vi "Retrieve.vi"(8 "error in (no error)":errorcluster, 11 "Error Code":i32) -> (0 "error out":errorcluster, 3 "Filter?":bool)   [LabVIEW 2026, in "TALOS.lvlib" / "Classes.lvlib" / "Error Filter.lvclass"]
doc: "Use this VI to add an error to be skipped in the future. If repetitions and time are both left to zero, the error will be permanently skipped: otherwise the error will be skipped until at least one of the two conditions will be met."
uses:
  Error Filter.lvclass
  Ancestor/Ancestor/Ancestor.lvclass/Ancestor.ctl
  Support VIs/Generate Error.vi
  FGV/Error Memory/Get Error Description.vi
  Support VIs/Get PC name.vi
  Ancestor/Ancestor/Read ID.vi
  Support VIs/Get Class Name.vi
  <vilib>/Utility/error.llb/Clear Errors.vi
  FGV/Error Memory/Error Memory Core.vi
  <vilib>/AdvancedString/Delimited String to 1D String Array.vi
  <vilib>/AdvancedString/Delimited String to 1D String Array (string).vi
  Support VIs/Circus Root Path.vi
  FGV/Error Memory/Error Crt Lvl checker.vi
  FGV/Error Memory/Error Memory Core.vi/40c8088d-b597-4017-91af-faa98e00292e.vi
  FGV/Error Memory/Error Memory Core.vi/d4a3ab98-063c-4e44-b43d-fbdcfe6c2be2.vi
  Support VIs/Global Memory.vi
  <vilib>/Utility/LVClass/Get LV Class Name.vi
  Support VIs/Is in Packed Library.vi
  Support VIs/TALOS Root path.vi
  Support VIs/Read CSV worksheet.vi
  Support VIs/Global Constants.vi
  <vilib>/Utility/error.llb/General Error Handler.vi
  Support VIs/Error Log.vi
  Ancestor/Ancestor/Ancestor.lvclass
  <vilib>/Comparison/Equal/Equal Functor/Equal Functor.lvclass
  TALOS.lvlib
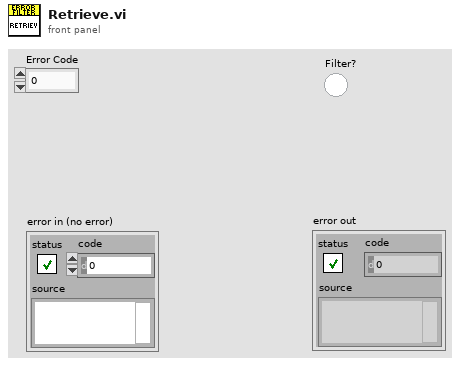
[diagram p1: front panel]
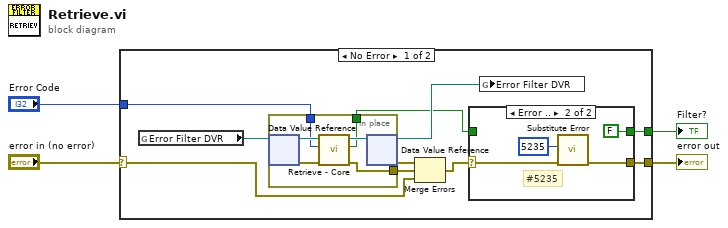
[diagram p0: block diagram]
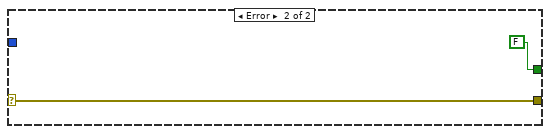
[diagram p3: hidden frame]
diagram:
  n1 = case shown="No Error" "error in (no error)" {
    selector: "error in (no error)" -> [w14 w28]
    tunnel: [w12 w28] -> w2
    tunnel: "Error Code" -> [w9 _]
    tunnel: [w7 FALSE ("Filter")] -> w1
    frame No Error {
      n2 = global read "Global Memory.vi" "Error Filter DVR"() -> (w11:refnum<data-value>)
      n3 = in-place {
        in-place-border: w9 -> [w16]
        in-place-border: [w17] -> w8
        in-place-border: [w15] -> w5
        n4 = in-place-dvr #1(w11) -> (w20:refnum<class "Error Filter.lvclass">, w18:errorcluster)
        n5 = call "Retrieve - Core.vi"("error in (no error)"=w18, "Error code"=w16, "Error Filter in"=w20) -> ("error out"=w17:errorcluster, "Filter"=w15:bool, "Error Filter out"=w19:refnum<class "Error Filter.lvclass">)  [unwired: 6 in]
        n6 = in-place-dvr #1(w19) -> (w6:refnum<data-value>, w10:errorcluster)
      }
      n7 = Merge Errors(w10, w8, w14) -> (w13:errorcluster)
      n8 = case shown="Error .." w13 {
        selector: w13 -> [w22 w26]
        tunnel: [w22 w25] -> w12
        tunnel: w5 -> [w21 _]
        tunnel: [w21 FALSE ("Filter")] -> w7
        frame No Error {
        }
        frame Error {
          # "#5235"
          n9 = call "Substitute Error.vi"("error in (no error)"=w26, "Error Code"=5235) -> ("error out"=w25:errorcluster)  [unwired: 9 in]
        }
      }
      n10 = global write "Global Memory.vi" "Error Filter DVR"(w6) -> ()
    }
    frame Error {
    }
  }
  "error out" <- w2
  "Filter?" <- w1
